vi "PumpValveHeaterStopproto.vi"() -> ()   [LabVIEW 2015]
uses:
  PumpValve.ctl
  <vilib>/DAQmx/read.llb/DAQmx Read (Analog 1D Wfm NChan 1Samp).vi
  <vilib>/DAQmx/write.llb/DAQmx Write (Digital 1D Bool NChan 1Samp 1Line).vi
  <vilib>/DAQmx/miscellaneous.llb/DAQmx Fill In Error Info.vi
  <vilib>/addons/control/pid/pid.llb/PID Advanced (DBL).vi
  <vilib>/addons/control/pid/NI_PID_pid.lvlib
panel:
  out "Pressure (mBar)":dbl format="%#_13g"
  out "Voltage Reading (Pressure)":dbl format="%#_13g"
  out "Pressure Chart Voltage":waveform(dbl)(graph)
  out "Voltage Reading(Temp)":dbl format="%#_13g"
  out "Temperature (Celcius)":dbl format="%#_13g"
  out "Temp(C)":dbl(slide) scale=-10.0..100.0
  out "Temp Chart":waveform(dbl)(graph)
  out "Duty Cycle from Control Value":dbl
  out "Control Value Pressure":dbl
  out "Heater On/off":bool
  out "Control Value (Temp Sensor)":dbl(knob) scale=0.0..100.0
  in  "PID gains Temp":T1={"proportional gain (Kc)"=1.0, "integral time (Ti, min)"=0.01, "derivative time (Td, min)"=0.0} {"derivative time (Td, min)" format="%.3f"; "integral time (Ti, min)" format="%.3f"; "proportional gain (Kc)" format="%.3f"}
  in  "Temp Setting":dbl
  in  "Maintain Temp":bool
  in  "Stop Maintaining Pressure":bool
  in  "PID gains":T1={"proportional gain (Kc)"=1.0, "integral time (Ti, min)"=0.01, "derivative time (Td, min)"=0.0} {"derivative time (Td, min)" format="%.3f"; "integral time (Ti, min)" format="%.3f"; "proportional gain (Kc)" format="%.3f"}
  out "Control Value (Pressure Sensor)":dbl(knob) scale=-10.0..10.0
  in  "Pressure Setting (mBar)":dbl
  in  "Maintain pressure":bool
  in  "On/Off Temp":bool
  in  "Manual Mode Temp":bool
  in  "Duty cycle % (0-100)":dbl=50.0
  in  "Steps in a cycle":i32=256
  in  "Cycle time (s)":dbl=5.0
  in  "On/Off (Pump)":bool
  in  "Open/Close (Blue)":bool
  in  "Open/Close (Green)":bool
  in  "Manual Mode Pump/Valve":bool
  out "Invalid fill%":bool
  out "Tank":u32(slide) scale=0.0..100.0
  in  "Drain %":u32
  in  "Fill %":u32
  in  "Drain":bool
  in  "Stop Program":bool
  in  "Fill":bool
  # "Temp only adjusts up (do nothing to cool?)"
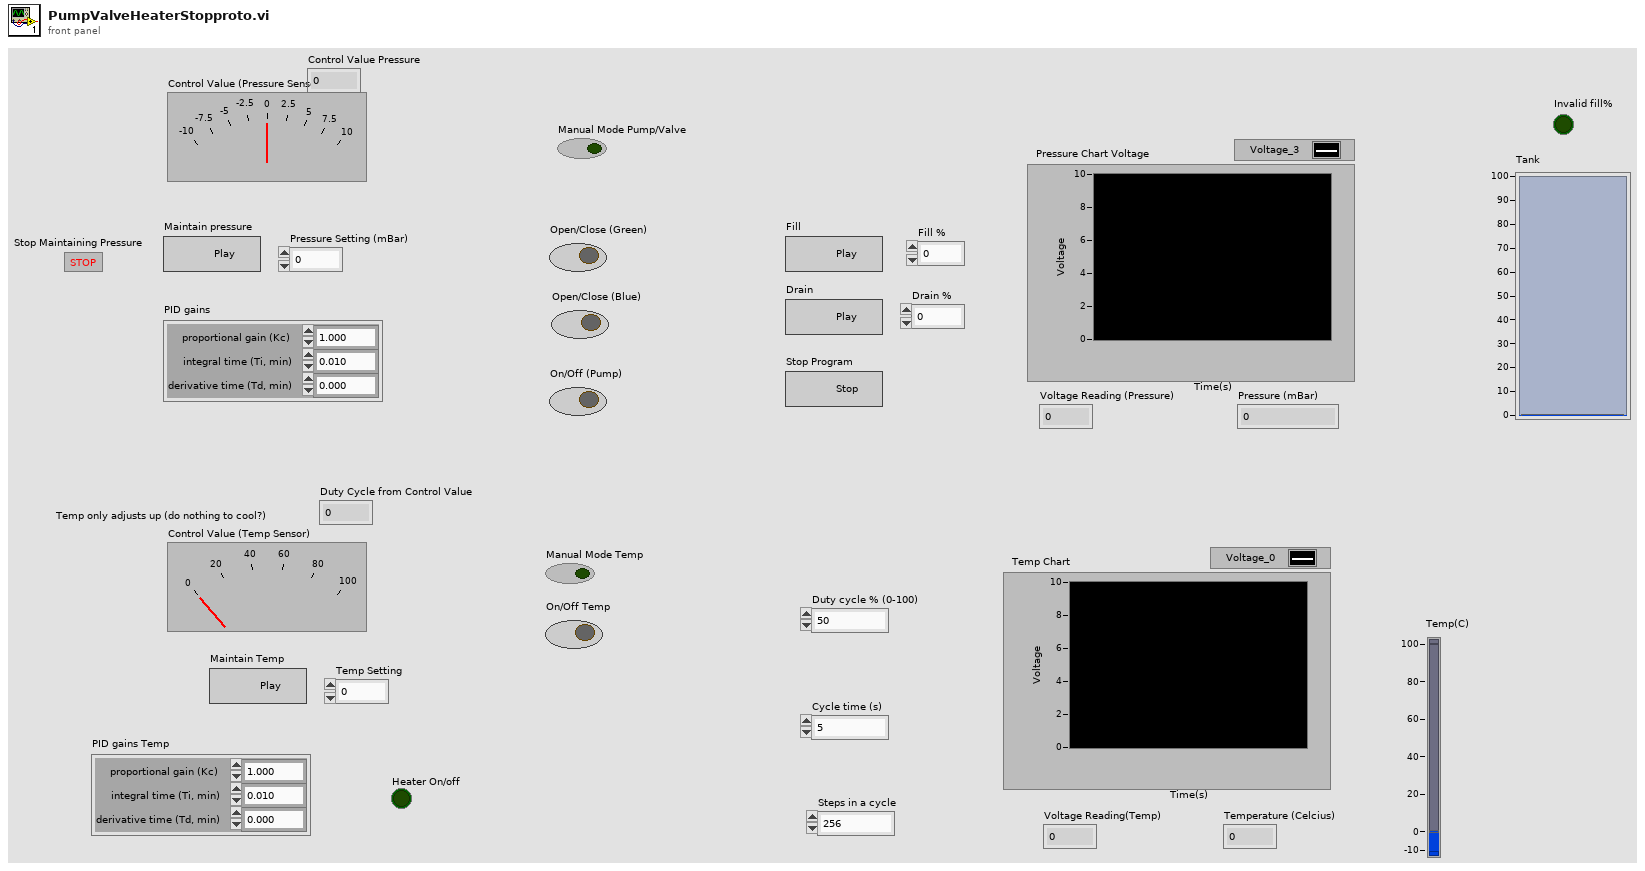
[diagram p1: front panel]
types:
  T1 = cluster{"proportional gain (Kc)":dbl, "integral time (Ti, min)":dbl, "derivative time (Td, min)":dbl}
  T2 = typedef "PumpValve.ctl" = enum16{"PressureSetting", "ManualPressure", "ManualTemp", "Idle Temp", "Set Temp", "Initialize", "Idle", "Fill", "Drain", "Stop"}
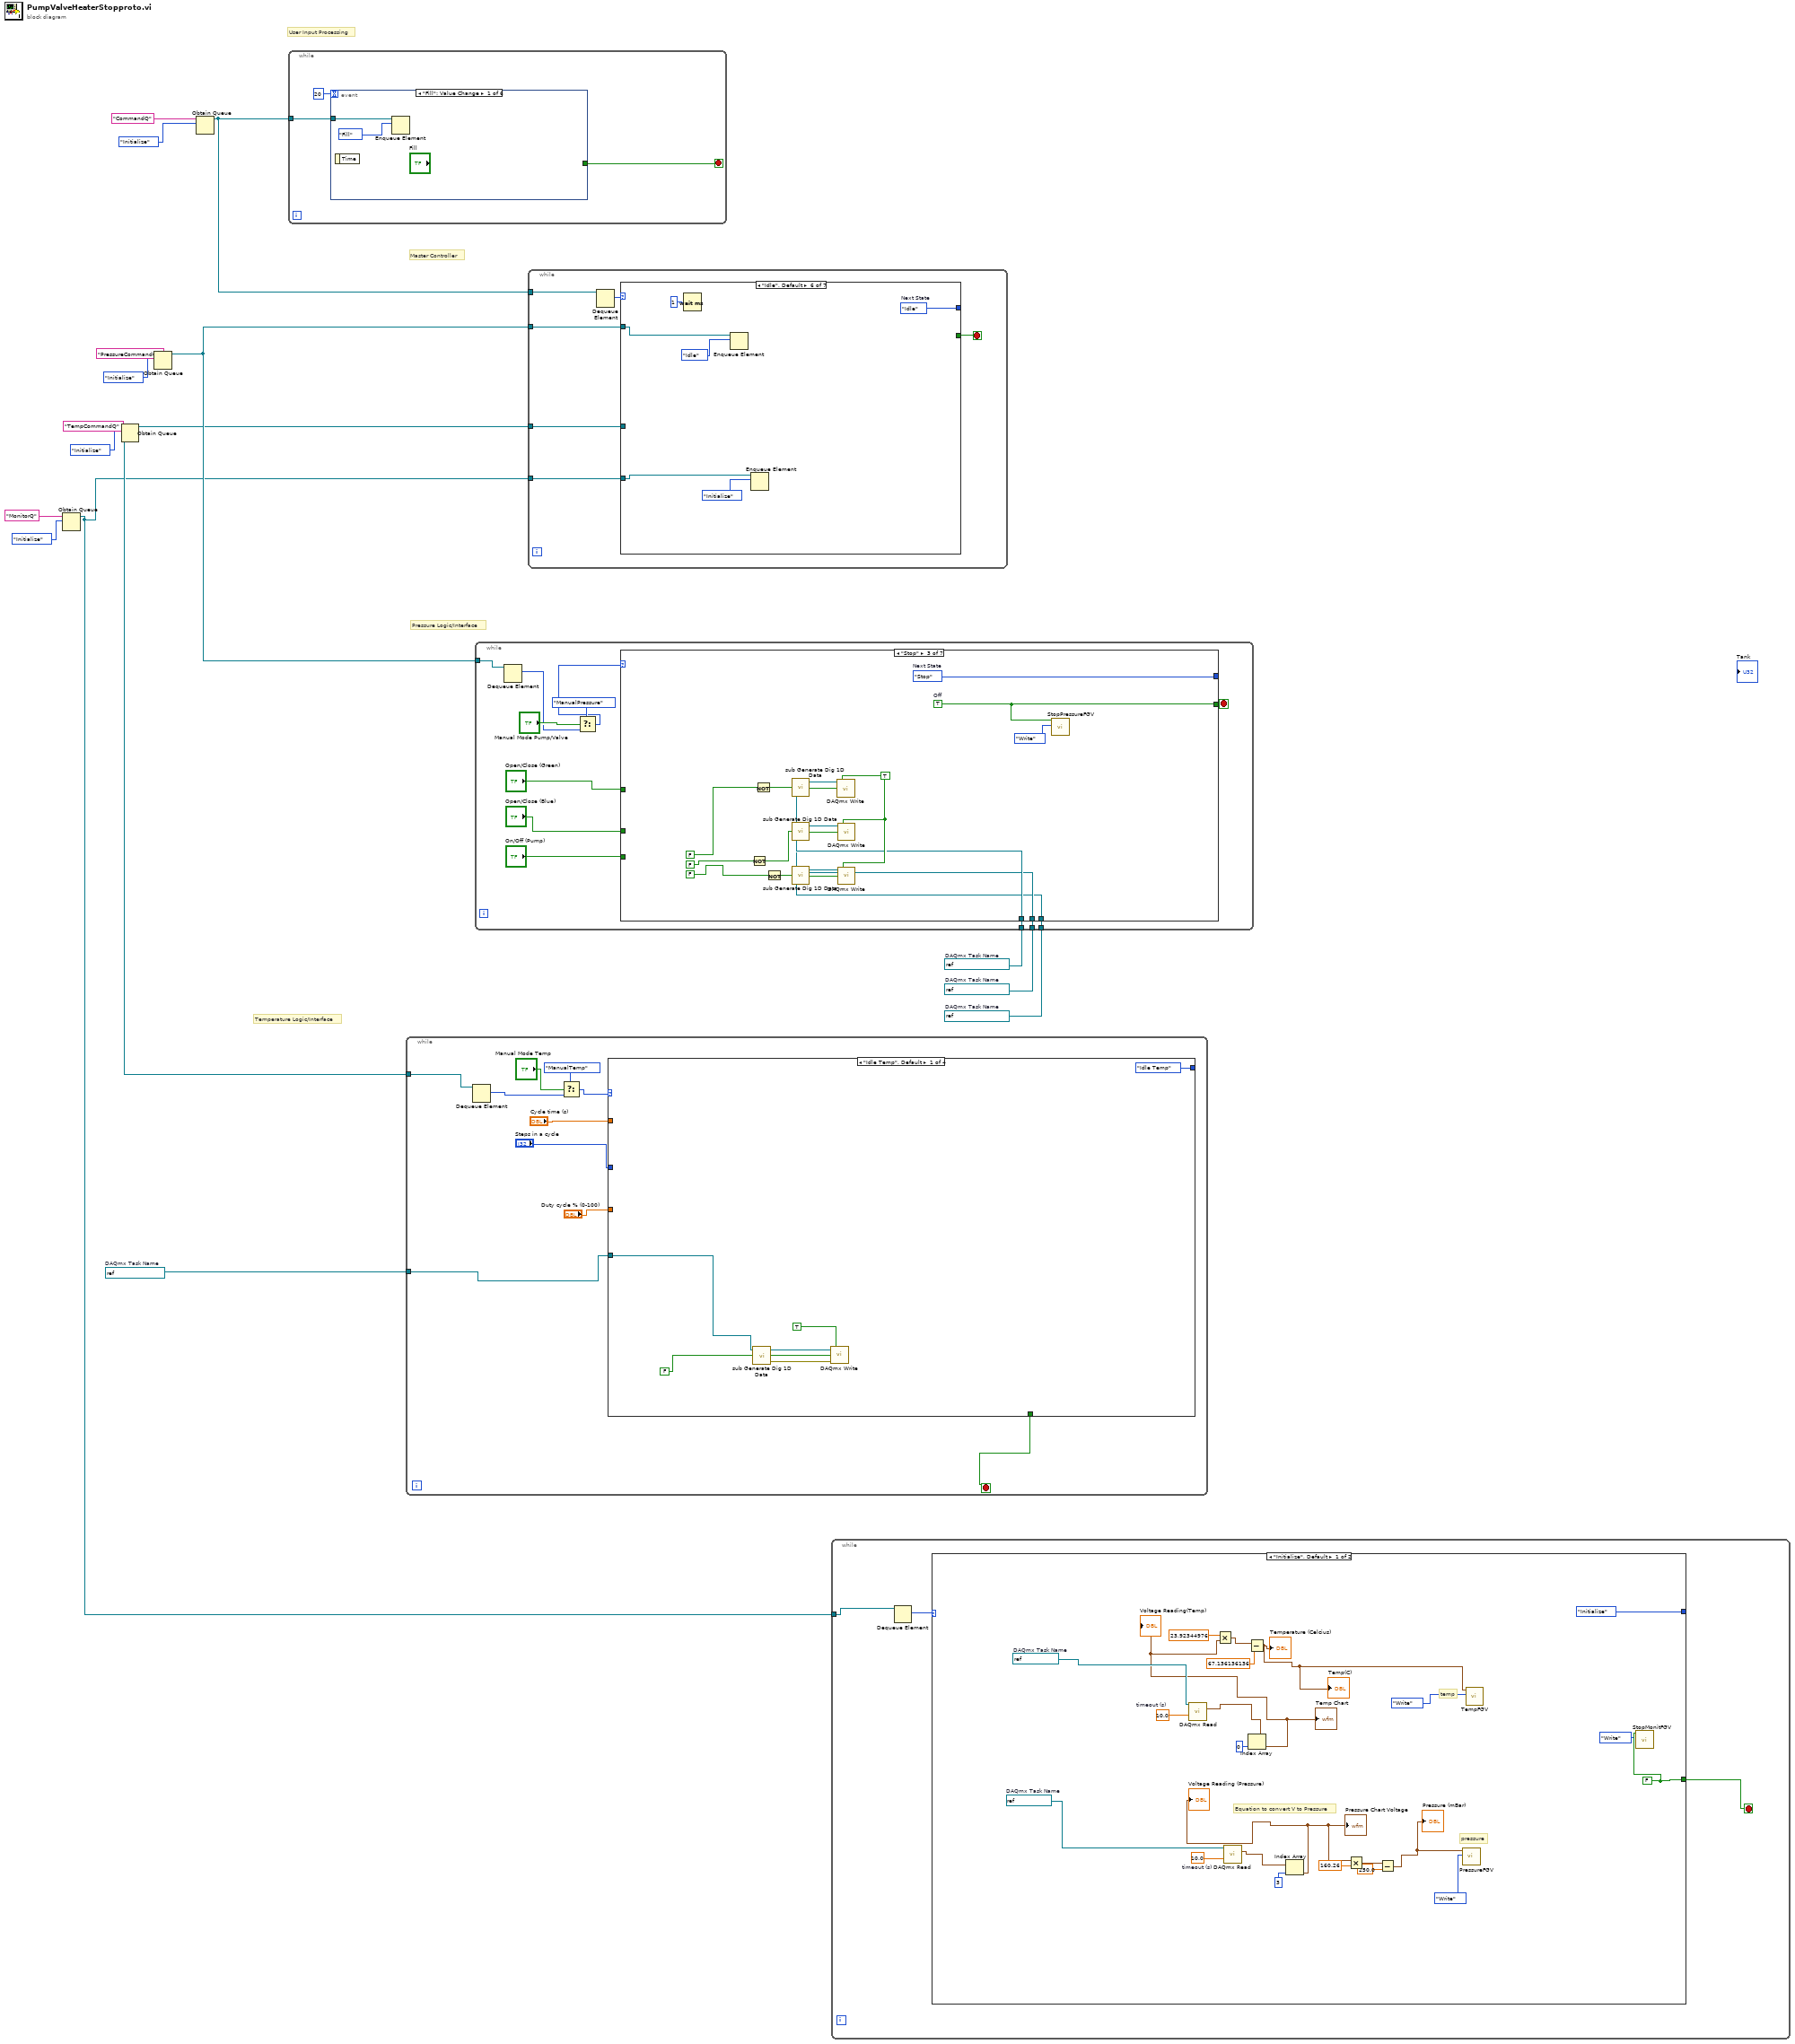
[diagram p0: block diagram]
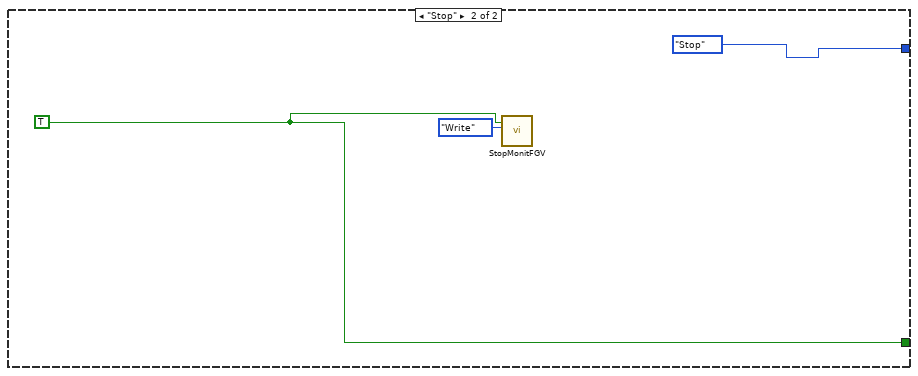
[diagram p2: hidden frame]
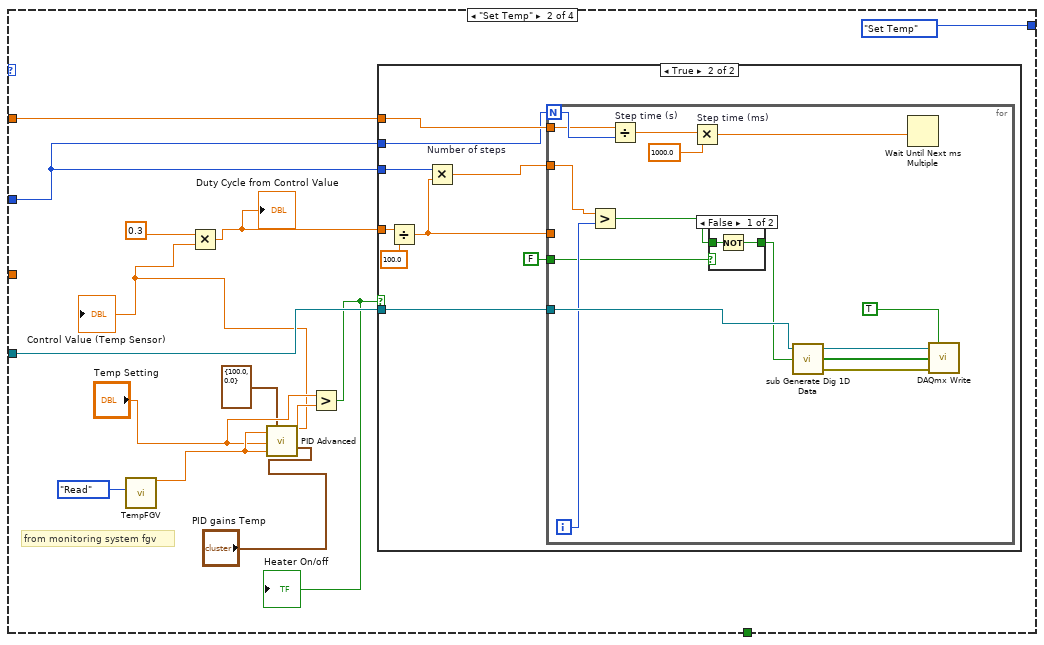
[diagram p3: hidden frame]
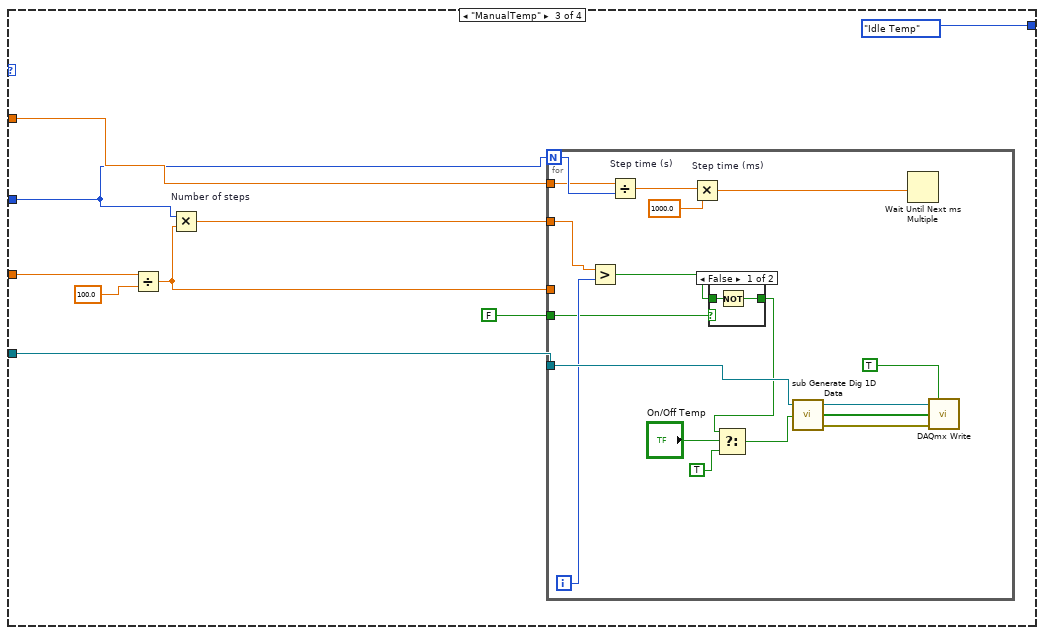
[diagram p6: hidden frame]
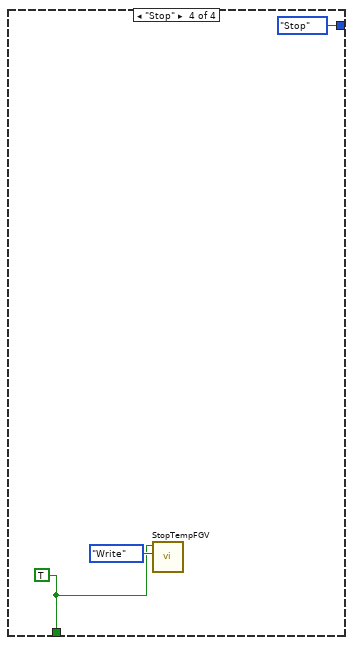
[diagram p8: hidden frame]
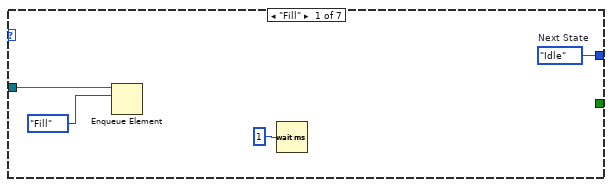
[diagram p9: hidden frame]
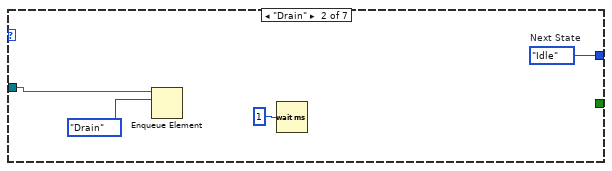
[diagram p10: hidden frame]
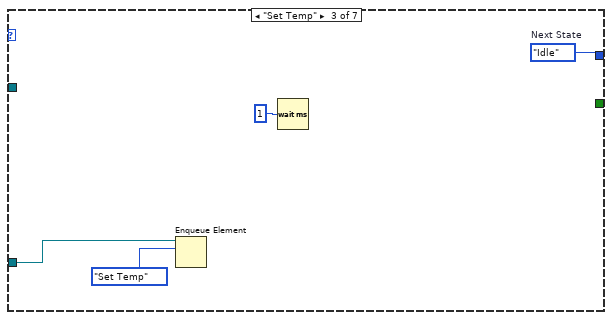
[diagram p11: hidden frame]
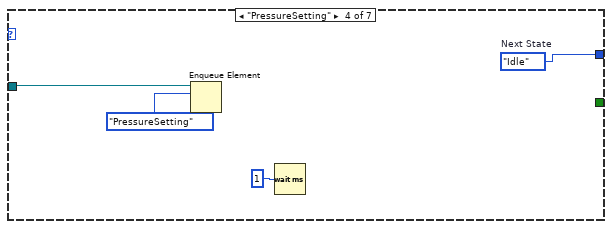
[diagram p12: hidden frame]
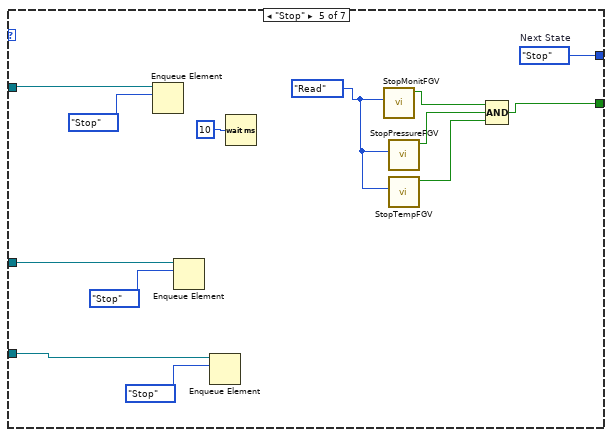
[diagram p13: hidden frame]
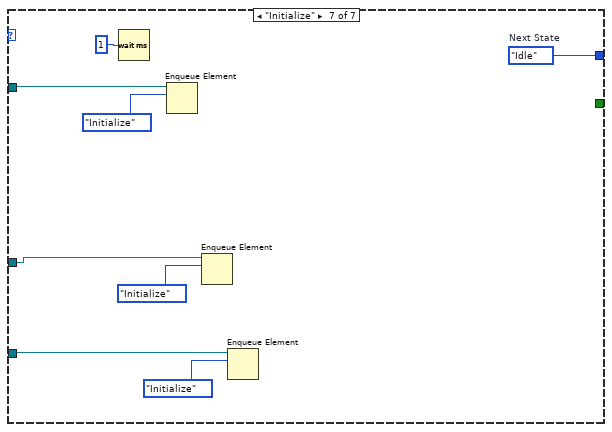
[diagram p14: hidden frame]
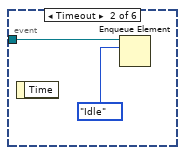
[diagram p15: hidden frame]
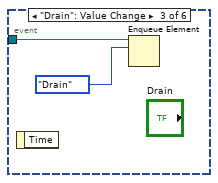
[diagram p16: hidden frame]
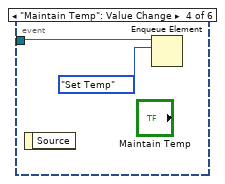
[diagram p17: hidden frame]
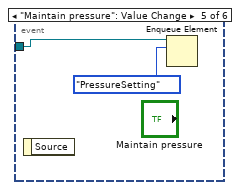
[diagram p18: hidden frame]
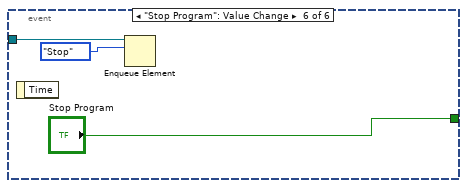
[diagram p19: hidden frame]
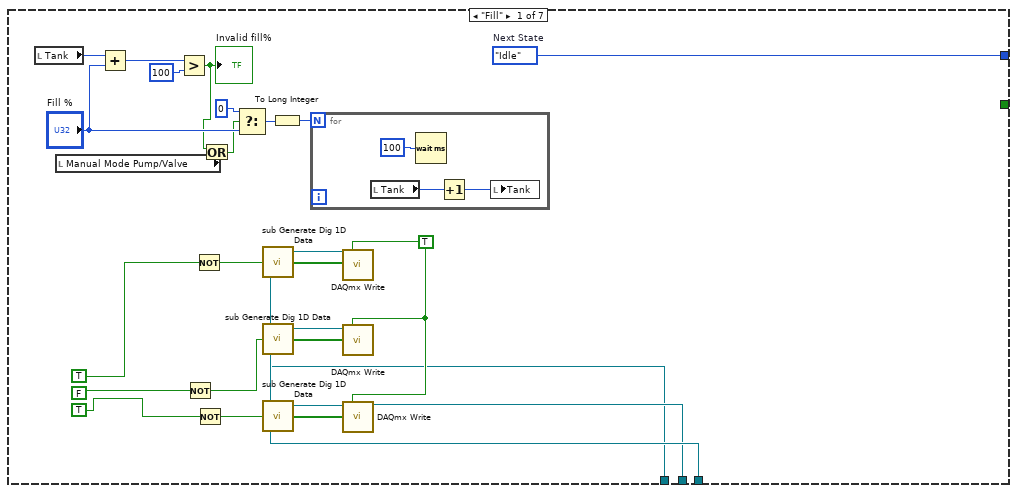
[diagram p20: hidden frame]
diagram:
  w7 = refnum<k21> "YellowdigOUT"  # DAQmx Task Name
  w12 = refnum<k21> "DigitalOutGreen"  # DAQmx Task Name
  w13 = refnum<k21> "DigitalOutGreen"  # DAQmx Task Name
  w14 = refnum<k21> "DigitalOutGreen"  # DAQmx Task Name
  # "Temperature Logic/Interface"
  # "Pressure Logic/Interface"
  # "Master Controller"
  # "User Input Processing"
  n1 = Obtain Queue(name (unnamed)="MonitorQ", element data type=PumpValve."Initialize" ("States")) -> (queue out=w1:refnum<queue>)  [unwired: 3 in, 2 out]
  n2 = Obtain Queue(name (unnamed)="TempCommandQ", element data type=PumpValve."Initialize" ("States")) -> (queue out=w4:refnum<queue>)  [unwired: 3 in, 2 out]
  n3 = Obtain Queue(name (unnamed)="PressureCommandQ", element data type=PumpValve."Initialize" ("States")) -> (queue out=w8:refnum<queue>)  [unwired: 3 in, 2 out]
  n4 = Obtain Queue(name (unnamed)="CommandQ", element data type=PumpValve."Initialize" ("States")) -> (queue out=w11:refnum<queue>)  [unwired: 3 in, 2 out]
  n5 = while {
    tunnel: w11 -> [w18]
    stop <- w17 stop-if-true
    n6 = event shown="[0] \"Fill\": Value Change" {
      selector: _ -> [_ _ _ _ _ _]
      dyn-events: _ -> [_ _ _ _ _ _]
      timeout: 20 -> [_ _ _ _ _ _]
      tunnel: w18 -> [w21 w23 w25 w26 w29 w32]
      tunnel: [_ _ _ _ _ "Stop Program"] -> w17
      event "Fill": Value Change {
        n7 = event-data() -> ()  [unwired: 1 in, 1 out]
        n8 = Enqueue Element(queue=w21, element=PumpValve."Fill" ("States")) -> ()  [unwired: 2 in, 3 out]
      }
      event Timeout {
        n9 = event-data() -> ()  [unwired: 1 in, 1 out]
        n10 = Enqueue Element(queue=w23, element=PumpValve."Idle" ("States")) -> ()  [unwired: 2 in, 3 out]
      }
      event "Drain": Value Change {
        n11 = event-data() -> ()  [unwired: 1 in, 1 out]
        n12 = Enqueue Element(queue=w25, element=PumpValve."Drain" ("States")) -> ()  [unwired: 2 in, 3 out]
      }
      event "Maintain Temp": Value Change {
        n13 = event-data() -> ()  [unwired: 1 in, 1 out]
        n14 = Enqueue Element(queue=w26, element=PumpValve."Set Temp" ("States")) -> ()  [unwired: 2 in, 3 out]
      }
      event "Maintain pressure": Value Change {
        n15 = event-data() -> ()  [unwired: 1 in, 1 out]
        n16 = Enqueue Element(queue=w29, element=PumpValve."PressureSetting" ("States")) -> ()  [unwired: 2 in, 3 out]
      }
      event "Stop Program": Value Change {
        n17 = event-data() -> ()  [unwired: 1 in, 1 out]
        n18 = Enqueue Element(queue=w32, element=PumpValve."Stop" ("States")) -> ()  [unwired: 2 in, 3 out]
      }
    }
  }
  n19 = while {
    tunnel: w7 -> [w42]
    tunnel: w4 -> [w41]
    stop <- w39 stop-if-true
    n20 = Dequeue Element(queue=w41) -> (element=w40:T2)  [unwired: 2 in, 3 out]
    n21 = Select(t=PumpValve."ManualTemp", s="Manual Mode Temp", f=w40) -> (s? t:f=w35:T2)
    n22 = case shown="\"Idle Temp\", Default" w35 {
      tunnel: w42 -> [w44 w62 w97 _]
      tunnel: [PumpValve."Idle Temp" ("States") PumpValve."Set Temp" ("States") PumpValve."Idle Temp" ("States") PumpValve."Stop" ("States")] -> _
      tunnel: "Cycle time (s)" -> [_ w60 w91 _]
      tunnel: "Steps in a cycle" -> [_ w59 w90 _]
      tunnel: "Duty cycle % (0-100)" -> [_ _ w89 _]
      tunnel: [_ _ _ w120] -> w39
      frame "Idle Temp", Default {
        n23 = call <vilib>:"sub Generate Dig 1D Data.vi"("initial value"=FALSE, "task in"=w44) -> ("error out"=w46:errorcluster, "Data"=w47:bool[], "task out"=w48:refnum<k21>)  [unwired: 1 in]
        n24 = call-poly <vilib>:"DAQmx Write.vi"("task/channels in"=w48, "auto start"=TRUE, "data"=w47, "error in"=w46) -> ()  [unwired: 9 in, 3 out]
      }
      frame "Set Temp" {
        # "from monitoring system fgv"
        n25 = call "TempFGV.vi"("Command"=enum16{"Write", "Read"}."Read") -> ("OUT"=w53:dbl)  [unwired: 10 in]
        n26 = call-poly <vilib>:"PID Advanced.vi"("setpoint"="Temp Setting", "output range"=cluster{"output high":dbl, "output low":dbl} {"output high"=100.0, "output low"=0.0}, "process variable"=w53, "PID gains"="PID gains Temp") -> ("output"=w51:dbl)  [unwired: 10 in, 1 out]
        "Control Value (Temp Sensor)" <- w51
        n27 = Multiply(x=0.3, y=w51) -> (x*y=w55:dbl)
        "Duty Cycle from Control Value" <- w55
        n28 = Greater?(x="Temp Setting", y=w53) -> (0:w58:bool)
        "Heater On/off" <- w58
        n29 = case shown="True" w58 {
          tunnel: w62 -> [_ w70]
          tunnel: w60 -> [_ w65]
          tunnel: w59 -> [_ w64]
          tunnel: w55 -> [_ w63]
          tunnel: w59 -> [_ _]
          frame False {
          }
          frame True {
            n30 = Divide(x=w63, y=100.0) -> (x/y=w68:dbl)
            n31 = Multiply "Number of steps"(x=w64, y=w68) -> (x*y=w67:dbl)
            n32 = for {
              N: w64 -> [w80]
              tunnel: w70 -> [w82]
              tunnel: w68 -> [_]
              tunnel: w65 -> [w79]
              tunnel: w67 -> [w75]
              tunnel: FALSE -> [w72]
              i -> [w74]
              n33 = Greater?(x=w75, y=w74) -> (0:w73:bool)
              n34 = Divide "Step time (s)"(x=w79, y=w80) -> (x/y=w78:dbl)
              n35 = Multiply "Step time (ms)"(x=w78, y=1000.0) -> (x*y=w76:dbl)
              n36 = case shown="False" w72 {
                tunnel: [w86 w88] -> w81
                tunnel: w73 -> [w87 w88]
                frame False {
                  n37 = Not(x=w87) -> (.not. x?=w86:bool)
                }
                frame True {
                }
              }
              n38 = call <vilib>:"sub Generate Dig 1D Data.vi"("initial value"=w81, "task in"=w82) -> ("error out"=w84:errorcluster, "Data"=w71:bool[], "task out"=w83:refnum<k21>)  [unwired: 1 in]
              n39 = Wait Until Next ms Multiple(millisecond multiple=w76) -> ()  [unwired: 1 out]
              n40 = call-poly <vilib>:"DAQmx Write.vi"("task/channels in"=w83, "auto start"=TRUE, "data"=w71, "error in"=w84) -> ()  [unwired: 9 in, 3 out]
            }
          }
        }
      }
      frame "ManualTemp" {
        n41 = Divide(x=w89, y=100.0) -> (x/y=w95:dbl)
        n42 = Multiply "Number of steps"(x=w90, y=w95) -> (x*y=w94:dbl)
        n43 = for {
          N: w90 -> [w110]
          tunnel: w97 -> [w111]
          tunnel: w95 -> [_]
          tunnel: w91 -> [w109]
          tunnel: w94 -> [w105]
          tunnel: FALSE -> [w102]
          i -> [w104]
          n44 = Greater?(x=w105, y=w104) -> (0:w103:bool)
          n45 = Divide "Step time (s)"(x=w109, y=w110) -> (x/y=w108:dbl)
          n46 = Multiply "Step time (ms)"(x=w108, y=1000.0) -> (x*y=w106:dbl)
          n47 = case shown="False" w102 {
            tunnel: [w116 w118] -> w100
            tunnel: w103 -> [w117 w118]
            frame False {
              n48 = Not(x=w117) -> (.not. x?=w116:bool)
            }
            frame True {
            }
          }
          n49 = Select(t=w100, s="On/Off Temp", f=TRUE) -> (s? t:f=w99:bool)
          n50 = call <vilib>:"sub Generate Dig 1D Data.vi"("initial value"=w99, "task in"=w111) -> ("error out"=w114:errorcluster, "Data"=w113:bool[], "task out"=w112:refnum<k21>)  [unwired: 1 in]
          n51 = Wait Until Next ms Multiple(millisecond multiple=w106) -> ()  [unwired: 1 out]
          n52 = call-poly <vilib>:"DAQmx Write.vi"("task/channels in"=w112, "auto start"=TRUE, "data"=w113, "error in"=w114) -> ()  [unwired: 9 in, 3 out]
        }
      }
      frame "Stop" {
        w120 = TRUE
        n53 = call "StopTempFGV.vi"("Command"=enum16{"Write", "Read"}."Write", "IN"=w120) -> ()  [unwired: 9 in, 1 out]
      }
    }
  }
  n54 = while {
    tunnel: w8 -> [w133]
    tunnel: w14 -> [w129]
    tunnel: w13 -> [w130]
    tunnel: w12 -> [w131]
    stop <- w132 stop-if-true
    n55 = Dequeue Element(queue=w133) -> (element=w126:T2)  [unwired: 2 in, 3 out]
    n56 = Select(t=PumpValve."ManualPressure", s="Manual Mode Pump/Valve", f=w126) -> (s? t:f=w125:T2)
    n57 = case shown="\"Stop\"" w125 {
      tunnel: [w160 w188 w210 w232 w252 w256 w302] -> _
      tunnel: [_ _ w193 _ _ _ _] -> w132
      tunnel: w131 -> [w142 w170 w200 w220 w240 w253 w291]
      tunnel: w130 -> [w141 w171 w201 w219 w239 w254 w292]
      tunnel: w129 -> [w140 w172 w202 w218 w238 w255 w293]
      tunnel: "Open/Close (Green)" -> [_ _ _ _ w235 _ _]
      tunnel: "Open/Close (Blue)" -> [_ _ _ _ w234 _ _]
      tunnel: "On/Off (Pump)" -> [_ _ _ _ w233 _ _]
      frame "Fill" {
        w149 = TRUE
        w160 = PumpValve."Idle"  # Next State
        n58 = local read "Tank"() -> (w159:u32)
        n59 = local read "Manual Mode Pump/Valve"() -> (w151:bool)
        n60 = Add(x=w159, y="Fill %") -> (x+y=w157:u32)
        n61 = Greater?(x=w157, y=u32 100) -> (0:w152:bool)
        "Invalid fill%" <- w152
        n62 = Not(x=FALSE) -> (.not. x?=w137:bool)
        n63 = Not(x=TRUE) -> (.not. x?=w138:bool)
        n64 = Not(x=TRUE) -> (.not. x?=w139:bool)
        n65 = Or(x=w152, y=w151) -> (x .or. y?=w150:bool)
        n66 = Select(t=u32 0, s=w150, f="Fill %") -> (s? t:f=w154:u32)
        n67 = call <vilib>:"sub Generate Dig 1D Data.vi"("initial value"=w138, "task in"=w140) -> ("Data"=w144:bool[], "task out"=w148:refnum<k21>)  [unwired: 1 in, 1 out]
        n68 = call <vilib>:"sub Generate Dig 1D Data.vi"("initial value"=w137, "task in"=w141) -> ("Data"=w145:bool[], "task out"=w147:refnum<k21>)  [unwired: 1 in, 1 out]
        n69 = call <vilib>:"sub Generate Dig 1D Data.vi"("initial value"=w139, "task in"=w142) -> ("Data"=w143:bool[], "task out"=w146:refnum<k21>)  [unwired: 1 in, 1 out]
        n70 = To Long Integer(number=w154) -> (32bit integer=w153:i32)
        n71 = for {
          N: w153 -> [_]
          n72 = local read "Tank"() -> (w163:u32)
          n73 = Wait (ms)(milliseconds to wait=u32 100 ("y")) -> ()  [unwired: 1 out]
          n74 = Increment(x=w163) -> (x+1=w162:u32)
          n75 = local write "Tank"(w162) -> ()
        }
        n76 = call-poly <vilib>:"DAQmx Write.vi"("task/channels in"=w148, "auto start"=w149, "data"=w144) -> ()  [unwired: 10 in, 3 out]
        n77 = call-poly <vilib>:"DAQmx Write.vi"("task/channels in"=w147, "auto start"=w149, "data"=w145) -> ()  [unwired: 10 in, 3 out]
        n78 = call-poly <vilib>:"DAQmx Write.vi"("task/channels in"=w146, "auto start"=w149, "data"=w143) -> ()  [unwired: 10 in, 3 out]
      }
      frame "Drain" {
        w173 = TRUE
        w188 = PumpValve."Idle"  # Next State
        n79 = local read "Tank"() -> (w185:u32)
        n80 = local read "Manual Mode Pump/Valve"() -> (w183:bool)
        n81 = Greater?(x="Drain %", y=w185) -> (0:w184:bool)
        n82 = Select(t=w185, s=w184, f="Drain %") -> (s? t:f=w187:u32)
        n83 = Not(x=FALSE) -> (.not. x?=w168:bool)
        n84 = Not(x=TRUE) -> (.not. x?=w167:bool)
        n85 = Not(x=TRUE) -> (.not. x?=w169:bool)
        n86 = To Long Integer(number=w187) -> (32bit integer=w180:i32)
        n87 = Select(t=0, s=w183, f=w180) -> (s? t:f=w181:i32)
        n88 = for {
          N: w181 -> [_]
          n89 = local read "Tank"() -> (w190:u32)
          n90 = Wait (ms)(milliseconds to wait=u32 100) -> ()  [unwired: 1 out]
          n91 = Decrement(x=w190) -> (x-1=w191:u32)
          n92 = local write "Tank"(w191) -> ()
        }
        n93 = call <vilib>:"sub Generate Dig 1D Data.vi"("initial value"=w168, "task in"=w172) -> ("Data"=w178:bool[], "task out"=w174:refnum<k21>)  [unwired: 1 in, 1 out]
        n94 = call <vilib>:"sub Generate Dig 1D Data.vi"("initial value"=w167, "task in"=w171) -> ("Data"=w177:bool[], "task out"=w175:refnum<k21>)  [unwired: 1 in, 1 out]
        n95 = call <vilib>:"sub Generate Dig 1D Data.vi"("initial value"=w169, "task in"=w170) -> ("Data"=w179:bool[], "task out"=w176:refnum<k21>)  [unwired: 1 in, 1 out]
        n96 = call-poly <vilib>:"DAQmx Write.vi"("task/channels in"=w174, "auto start"=w173, "data"=w178) -> ()  [unwired: 10 in, 3 out]
        n97 = call-poly <vilib>:"DAQmx Write.vi"("task/channels in"=w175, "auto start"=w173, "data"=w177) -> ()  [unwired: 10 in, 3 out]
        n98 = call-poly <vilib>:"DAQmx Write.vi"("task/channels in"=w176, "auto start"=w173, "data"=w179) -> ()  [unwired: 10 in, 3 out]
      }
      frame "Stop" {
        w209 = TRUE
        w193 = TRUE  # Off
        w210 = PumpValve."Stop"  # Next State
        n99 = Not(x=FALSE) -> (.not. x?=w197:bool)
        n100 = Not(x=FALSE) -> (.not. x?=w198:bool)
        n101 = Not(x=FALSE) -> (.not. x?=w199:bool)
        n102 = call <vilib>:"sub Generate Dig 1D Data.vi"("initial value"=w198, "task in"=w202) -> ("Data"=w204:bool[], "task out"=w208:refnum<k21>)  [unwired: 1 in, 1 out]
        n103 = call <vilib>:"sub Generate Dig 1D Data.vi"("initial value"=w197, "task in"=w201) -> ("Data"=w205:bool[], "task out"=w207:refnum<k21>)  [unwired: 1 in, 1 out]
        n104 = call <vilib>:"sub Generate Dig 1D Data.vi"("initial value"=w199, "task in"=w200) -> ("Data"=w203:bool[], "task out"=w206:refnum<k21>)  [unwired: 1 in, 1 out]
        n105 = call-poly <vilib>:"DAQmx Write.vi"("task/channels in"=w208, "auto start"=w209, "data"=w204) -> ()  [unwired: 10 in, 3 out]
        n106 = call-poly <vilib>:"DAQmx Write.vi"("task/channels in"=w207, "auto start"=w209, "data"=w205) -> ()  [unwired: 10 in, 3 out]
        n107 = call-poly <vilib>:"DAQmx Write.vi"("task/channels in"=w206, "auto start"=w209, "data"=w203) -> ()  [unwired: 10 in, 3 out]
        n108 = call "StopPressureFGV.vi"("Command"=enum16{"Write", "Read"}."Write", "IN"=w193) -> ()  [unwired: 9 in, 1 out]
      }
      frame "Idle", Default {
        w232 = PumpValve."Idle"  # Next State
        n109 = Wait (ms)(milliseconds to wait=u32 10) -> ()  [unwired: 1 out]
        n110 = Not(x=FALSE) -> (.not. x?=w216:bool)
        n111 = Not(x=FALSE) -> (.not. x?=w217:bool)
        n112 = Not(x=FALSE) -> (.not. x?=w223:bool)
        n113 = call <vilib>:"sub Generate Dig 1D Data.vi"("initial value"=w217, "task in"=w218) -> ("Data"=w225:bool[], "task out"=w229:refnum<k21>)  [unwired: 1 in, 1 out]
        n114 = call <vilib>:"sub Generate Dig 1D Data.vi"("initial value"=w216, "task in"=w219) -> ("Data"=w226:bool[], "task out"=w228:refnum<k21>)  [unwired: 1 in, 1 out]
        n115 = call <vilib>:"sub Generate Dig 1D Data.vi"("initial value"=w223, "task in"=w220) -> ("Data"=w224:bool[], "task out"=w227:refnum<k21>)  [unwired: 1 in, 1 out]
        n116 = call-poly <vilib>:"DAQmx Write.vi"("task/channels in"=w229, "auto start"=TRUE, "data"=w225) -> ()  [unwired: 10 in, 3 out]
        n117 = call-poly <vilib>:"DAQmx Write.vi"("task/channels in"=w228, "auto start"=TRUE, "data"=w226) -> ()  [unwired: 10 in, 3 out]
        n118 = call-poly <vilib>:"DAQmx Write.vi"("task/channels in"=w227, "auto start"=TRUE, "data"=w224) -> ()  [unwired: 10 in, 3 out]
        n119 = call "StopPressureFGV.vi"("Command"=enum16{"Write", "Read"}."Write", "IN"=FALSE) -> ()  [unwired: 9 in, 1 out]
      }
      frame "ManualPressure" {
        w252 = PumpValve."Idle"  # Next State
        n120 = Wait (ms)(milliseconds to wait=u32 10) -> ()  [unwired: 1 out]
        n121 = Not(x=w234) -> (.not. x?=w236:bool)
        n122 = Not(x=w235) -> (.not. x?=w237:bool)
        n123 = Not(x=w233) -> (.not. x?=w243:bool)
        n124 = call <vilib>:"sub Generate Dig 1D Data.vi"("initial value"=w237, "task in"=w238) -> ("Data"=w245:bool[], "task out"=w249:refnum<k21>)  [unwired: 1 in, 1 out]
        n125 = call <vilib>:"sub Generate Dig 1D Data.vi"("initial value"=w236, "task in"=w239) -> ("Data"=w246:bool[], "task out"=w248:refnum<k21>)  [unwired: 1 in, 1 out]
        n126 = call <vilib>:"sub Generate Dig 1D Data.vi"("initial value"=w243, "task in"=w240) -> ("Data"=w244:bool[], "task out"=w247:refnum<k21>)  [unwired: 1 in, 1 out]
        n127 = call-poly <vilib>:"DAQmx Write.vi"("task/channels in"=w249, "auto start"=TRUE, "data"=w245) -> ()  [unwired: 10 in, 3 out]
        n128 = call-poly <vilib>:"DAQmx Write.vi"("task/channels in"=w248, "auto start"=TRUE, "data"=w246) -> ()  [unwired: 10 in, 3 out]
        n129 = call-poly <vilib>:"DAQmx Write.vi"("task/channels in"=w247, "auto start"=TRUE, "data"=w244) -> ()  [unwired: 10 in, 3 out]
      }
      frame "PressureSetting" {
        w256 = PumpValve."Idle"  # Next State
        n130 = while {
          tunnel: w255 -> [w260]
          tunnel: w254 -> [w259]
          tunnel: w253 -> [w258]
          stop <- "Stop Maintaining Pressure" stop-if-true
          # "config for pump/valve"
          # "from monitoring system"
          # "output to hardware"
          n131 = call "PressureFGV.vi"("Command"=enum16{"Write", "Read"}."Read") -> ("OUT"=w277:dbl)  [unwired: 10 in]
          n132 = call-poly <vilib>:"PID Advanced.vi"("setpoint"="Pressure Setting (mBar)", "output range"=cluster{"output high":dbl, "output low":dbl} {"output high"=10.0, "output low"=-10.0}, "process variable"=w277, "PID gains"="PID gains") -> ("output"=w274:dbl)  [unwired: 10 in, 1 out]
          "Control Value (Pressure Sensor)" <- w274
          "Control Value Pressure" <- w274
          n133 = Greater?(x=w274, y=0.0) -> (0:w257:bool)
          n134 = Not(x=w257) -> (.not. x?=w261:bool)
          n135 = Not(x=w257) -> (.not. x?=w262:bool)
          n136 = Not(x=w257) -> (.not. x?=w265:bool)
          n137 = call <vilib>:"sub Generate Dig 1D Data.vi"("initial value"=w262, "task in"=w260) -> ("Data"=w267:bool[], "task out"=w271:refnum<k21>)  [unwired: 1 in, 1 out]
          n138 = call <vilib>:"sub Generate Dig 1D Data.vi"("initial value"=w261, "task in"=w259) -> ("Data"=w268:bool[], "task out"=w270:refnum<k21>)  [unwired: 1 in, 1 out]
          n139 = call <vilib>:"sub Generate Dig 1D Data.vi"("initial value"=w265, "task in"=w258) -> ("Data"=w266:bool[], "task out"=w269:refnum<k21>)  [unwired: 1 in, 1 out]
          n140 = call-poly <vilib>:"DAQmx Write.vi"("task/channels in"=w271, "auto start"=TRUE, "data"=w267) -> ()  [unwired: 10 in, 3 out]
          n141 = call-poly <vilib>:"DAQmx Write.vi"("task/channels in"=w270, "auto start"=TRUE, "data"=w268) -> ()  [unwired: 10 in, 3 out]
          n142 = call-poly <vilib>:"DAQmx Write.vi"("task/channels in"=w269, "auto start"=TRUE, "data"=w266) -> ()  [unwired: 10 in, 3 out]
        }
      }
      frame "Initialize" {
        w302 = PumpValve."Idle"  # Next State
        n143 = Wait (ms)(milliseconds to wait=u32 1) -> ()  [unwired: 1 out]
        n144 = Not(x=FALSE) -> (.not. x?=w287:bool)
        n145 = Not(x=FALSE) -> (.not. x?=w286:bool)
        n146 = Not(x=FALSE) -> (.not. x?=w290:bool)
        n147 = call <vilib>:"sub Generate Dig 1D Data.vi"("initial value"=w287, "task in"=w293) -> ("Data"=w295:bool[], "task out"=w299:refnum<k21>)  [unwired: 1 in, 1 out]
        n148 = call <vilib>:"sub Generate Dig 1D Data.vi"("initial value"=w286, "task in"=w292) -> ("Data"=w296:bool[], "task out"=w298:refnum<k21>)  [unwired: 1 in, 1 out]
        n149 = call <vilib>:"sub Generate Dig 1D Data.vi"("initial value"=w290, "task in"=w291) -> ("Data"=w294:bool[], "task out"=w297:refnum<k21>)  [unwired: 1 in, 1 out]
        n150 = call-poly <vilib>:"DAQmx Write.vi"("task/channels in"=w299, "auto start"=TRUE, "data"=w295) -> ()  [unwired: 10 in, 3 out]
        n151 = call-poly <vilib>:"DAQmx Write.vi"("task/channels in"=w298, "auto start"=TRUE, "data"=w296) -> ()  [unwired: 10 in, 3 out]
        n152 = call-poly <vilib>:"DAQmx Write.vi"("task/channels in"=w297, "auto start"=TRUE, "data"=w294) -> ()  [unwired: 10 in, 3 out]
        n153 = call "StopPressureFGV.vi"("Command"=enum16{"Write", "Read"}."Write", "IN"=FALSE) -> ()  [unwired: 9 in, 1 out]
      }
    }
  }
  n154 = while {
    tunnel: w11 -> [w307]
    tunnel: w8 -> [w306]
    tunnel: w4 -> [w304]
    tunnel: w1 -> [w303]
    stop <- w305 stop-if-true
    n155 = Dequeue Element(queue=w307) -> (element=w308:T2)  [unwired: 2 in, 3 out]
    n156 = case shown="\"Idle\", Default" w308 {
      tunnel: [w312 w316 w318 w322 w337 w343 w351] -> _
      tunnel: w306 -> [w309 w313 _ w321 w334 w340 w348]
      tunnel: [_ _ _ _ w329 _ _] -> w305
      tunnel: w304 -> [_ _ w317 _ w332 _ w345]
      tunnel: w303 -> [_ _ _ _ w330 w338 w344]
      frame "Fill" {
        w312 = PumpValve."Idle"  # Next State
        n157 = Enqueue Element(queue=w309, element=PumpValve."Fill" ("States")) -> ()  [unwired: 2 in, 3 out]
        n158 = Wait (ms)(milliseconds to wait=u32 1) -> ()  [unwired: 1 out]
      }
      frame "Drain" {
        w316 = PumpValve."Idle"  # Next State
        n159 = Enqueue Element(queue=w313, element=PumpValve."Drain" ("States")) -> ()  [unwired: 2 in, 3 out]
        n160 = Wait (ms)(milliseconds to wait=u32 1) -> ()  [unwired: 1 out]
      }
      frame "Set Temp" {
        w318 = PumpValve."Idle"  # Next State
        n161 = Enqueue Element(queue=w317, element=PumpValve."Set Temp" ("States")) -> ()  [unwired: 2 in, 3 out]
        n162 = Wait (ms)(milliseconds to wait=u32 1) -> ()  [unwired: 1 out]
      }
      frame "PressureSetting" {
        w322 = PumpValve."Idle"  # Next State
        n163 = Enqueue Element(queue=w321, element=PumpValve."PressureSetting" ("States")) -> ()  [unwired: 2 in, 3 out]
        n164 = Wait (ms)(milliseconds to wait=u32 1) -> ()  [unwired: 1 out]
      }
      frame "Stop" {
        w328 = enum16{"Write", "Read"}."Read" ("Command")
        w337 = PumpValve."Stop"  # Next State
        n165 = Enqueue Element(queue=w334, element=PumpValve."Stop" ("States")) -> ()  [unwired: 2 in, 3 out]
        n166 = Enqueue Element(queue=w332, element=PumpValve."Stop" ("States")) -> ()  [unwired: 2 in, 3 out]
        n167 = Enqueue Element(queue=w330, element=PumpValve."Stop" ("States")) -> ()  [unwired: 2 in, 3 out]
        n168 = Wait (ms)(milliseconds to wait=u32 10) -> ()  [unwired: 1 out]
        n169 = call "StopMonitFGV.vi"("Command"=w328) -> ("OUT"=w327:bool)  [unwired: 10 in]
        n170 = call "StopPressureFGV.vi"("Command"=w328) -> ("OUT"=w326:bool)  [unwired: 10 in]
        n171 = call "StopTempFGV.vi"("Command"=w328) -> ("OUT"=w325:bool)  [unwired: 10 in]
        n172 = Compound Arithmetic op=AND(w327, w326, w325) -> (w329:bool)
      }
      frame "Idle", Default {
        w343 = PumpValve."Idle"  # Next State
        n173 = Wait (ms)(milliseconds to wait=u32 1) -> ()  [unwired: 1 out]
        n174 = Enqueue Element(queue=w340, element=PumpValve."Idle" ("States")) -> ()  [unwired: 2 in, 3 out]
        n175 = Enqueue Element(queue=w338, element=PumpValve."Initialize" ("States")) -> ()  [unwired: 2 in, 3 out]
      }
      frame "Initialize" {
        w351 = PumpValve."Idle"  # Next State
        n176 = Wait (ms)(milliseconds to wait=u32 1) -> ()  [unwired: 1 out]
        n177 = Enqueue Element(queue=w348, element=PumpValve."Initialize" ("States")) -> ()  [unwired: 2 in, 3 out]
        n178 = Enqueue Element(queue=w345, element=PumpValve."Initialize" ("States")) -> ()  [unwired: 2 in, 3 out]
        n179 = Enqueue Element(queue=w344, element=PumpValve."Initialize" ("States")) -> ()  [unwired: 2 in, 3 out]
      }
    }
  }
  n180 = while {
    tunnel: w1 -> [w354]
    stop <- w352 stop-if-true
    n181 = Dequeue Element(queue=w354) -> (element=w353:T2)  [unwired: 2 in, 3 out]
    n182 = case shown="\"Initialize\", Default" w353 {
      tunnel: [w375 w379] -> w352
      tunnel: [PumpValve."Initialize" ("States") PumpValve."Stop" ("States")] -> _
      frame "Initialize", Default {
        w367 = 10.0  # timeout (s)
        w373 = 10.0  # timeout (s)
        w376 = refnum<k21> "AllAnalog"  # DAQmx Task Name
        w377 = refnum<k21> "AllAnalog"  # DAQmx Task Name
        w375 = FALSE
        # "Equation to convert V to Pressure"
        # "pressure"
        # "temp"
        n183 = call-poly <vilib>:"DAQmx Read.vi"("task/channels in"=w377, "timeout"=w373) -> ("data"=w364:waveform(dbl)[])  [unwired: 11 in, 2 out]
        n184 = call-poly <vilib>:"DAQmx Read.vi"("task/channels in"=w376, "timeout"=w367) -> ("data"=w361:waveform(dbl)[])  [unwired: 11 in, 2 out]
        n185 = Index Array(array=w364, index=0) -> (element=w363:waveform(dbl))
        "Voltage Reading(Temp)" <- w363
        "Temp Chart" <- w363
        n186 = Multiply(x=23.92344976, y=w363) -> (x*y=w371:waveform(dbl))
        n187 = Subtract(x=w371, y=67.136136136) -> (x-y=w368:waveform(dbl))
        "Temperature (Celcius)" <- w368
        "Temp(C)" <- w368
        n188 = Index Array(array=w361, index=3) -> (element=w360:waveform(dbl))
        "Pressure Chart Voltage" <- w360
        "Voltage Reading (Pressure)" <- w360
        n189 = Multiply(x=w360, y=160.26) -> (x*y=w358:waveform(dbl))
        n190 = Subtract(x=w358, y=250.0) -> (x-y=w356:waveform(dbl))
        "Pressure (mBar)" <- w356
        n191 = call "PressureFGV.vi"("Command"=enum16{"Write", "Read"}."Write", "IN"=w356) -> ()  [unwired: 9 in, 1 out]
        n192 = call "TempFGV.vi"("Command"=enum16{"Write", "Read"}."Write", "IN"=w368) -> ()  [unwired: 9 in, 1 out]
        n193 = call "StopMonitFGV.vi"("Command"=enum16{"Write", "Read"}."Write", "IN"=w375) -> ()  [unwired: 9 in, 1 out]
      }
      frame "Stop" {
        w379 = TRUE
        n194 = call "StopMonitFGV.vi"("Command"=enum16{"Write", "Read"}."Write", "IN"=w379) -> ()  [unwired: 9 in, 1 out]
      }
    }
  }
